vi "HH_Set.vi"(0 "Device List":T3(array[cluster]), 5 "CFD Settings":T2, 11 "error in (no error)":errorcluster, 12 "SyncDiv":i32, 13 "Offset":i32) -> (3 "ht3 header out":T1, 6 "Resolution (ps)":dbl, 8 "Range":i32, 10 "Sync Rate":i32, 15 "error out":errorcluster)   [LabVIEW 2009]
uses:
  CoreSetupNew/MT Scan/SubVIs/hhlib.dll
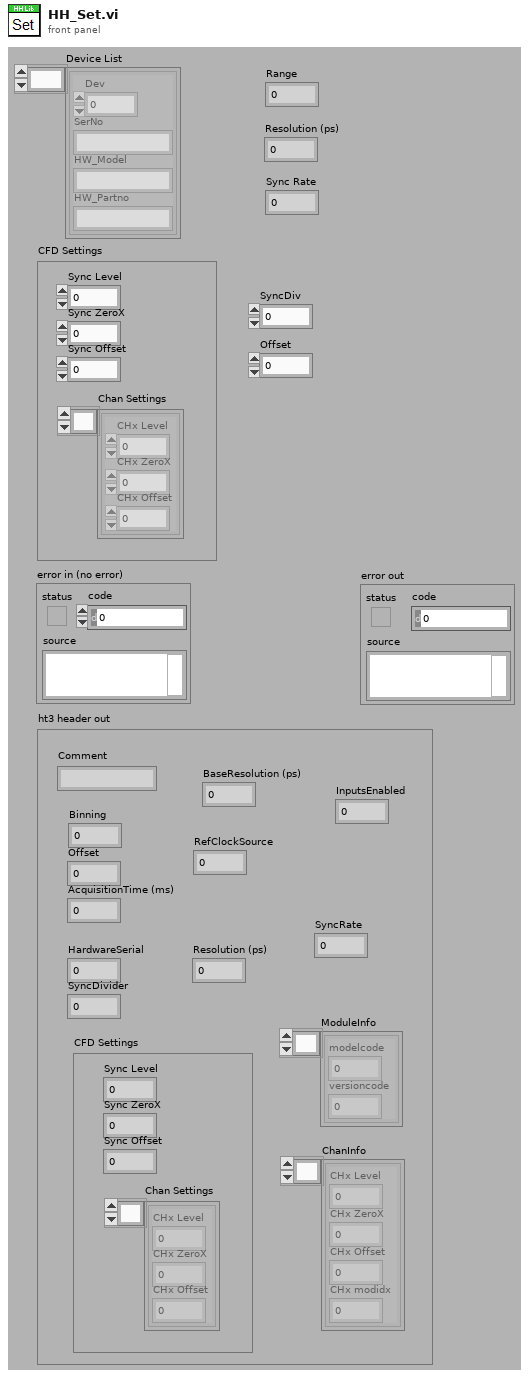
[diagram p1: front panel]
types:
  T1 = cluster{"Comment":string, "Binning":i32, "Offset":i32, "AcquisitionTime (ms)":i32, "HardwareSerial":i32, "SyncDivider":i32, "Resolution (ps)":dbl, "CFD Settings":cluster{"Sync Level":i32, "Sync ZeroX":i32, "Sync Offset":i32, "Chan Settings":cluster{"CHx Level":i32, "CHx ZeroX":i32, "CHx Offset":i32}[]}, "ModuleInfo":cluster{"modelcode":i32, "versioncode":i32}[], "BaseResolution (ps)":dbl, "RefClockSource":i32, "ChanInfo":cluster{"CHx Level":i32, "CHx ZeroX":i32, "CHx Offset":i32, "CHx modidx":i32}[], "SyncRate":i32, "InputsEnabled":i64}
  T2 = cluster{"Sync Level":i32, "Sync ZeroX":i32, "Sync Offset":i32, "Chan Settings":cluster{"CHx Level":i32, "CHx ZeroX":i32, "CHx Offset":i32}[]}
  T3 = cluster{"Dev":i32, "SerNo":string, "HW_Model":string, "HW_Partno":string}[]
  T4 = cluster{"CHx Level":i32, "CHx ZeroX":i32, "CHx Offset":i32, "CHx modidx":i32}
  T5 = cluster{"CHx Level":i32, "CHx ZeroX":i32, "CHx Offset":i32}
  T6 = cluster{"CHx Level":i32, "CHx ZeroX":i32, "CHx Offset":i32, "CHx modidx":i32}[]
  T7 = cluster{"CHx Level":i32, "CHx ZeroX":i32, "CHx Offset":i32}[]
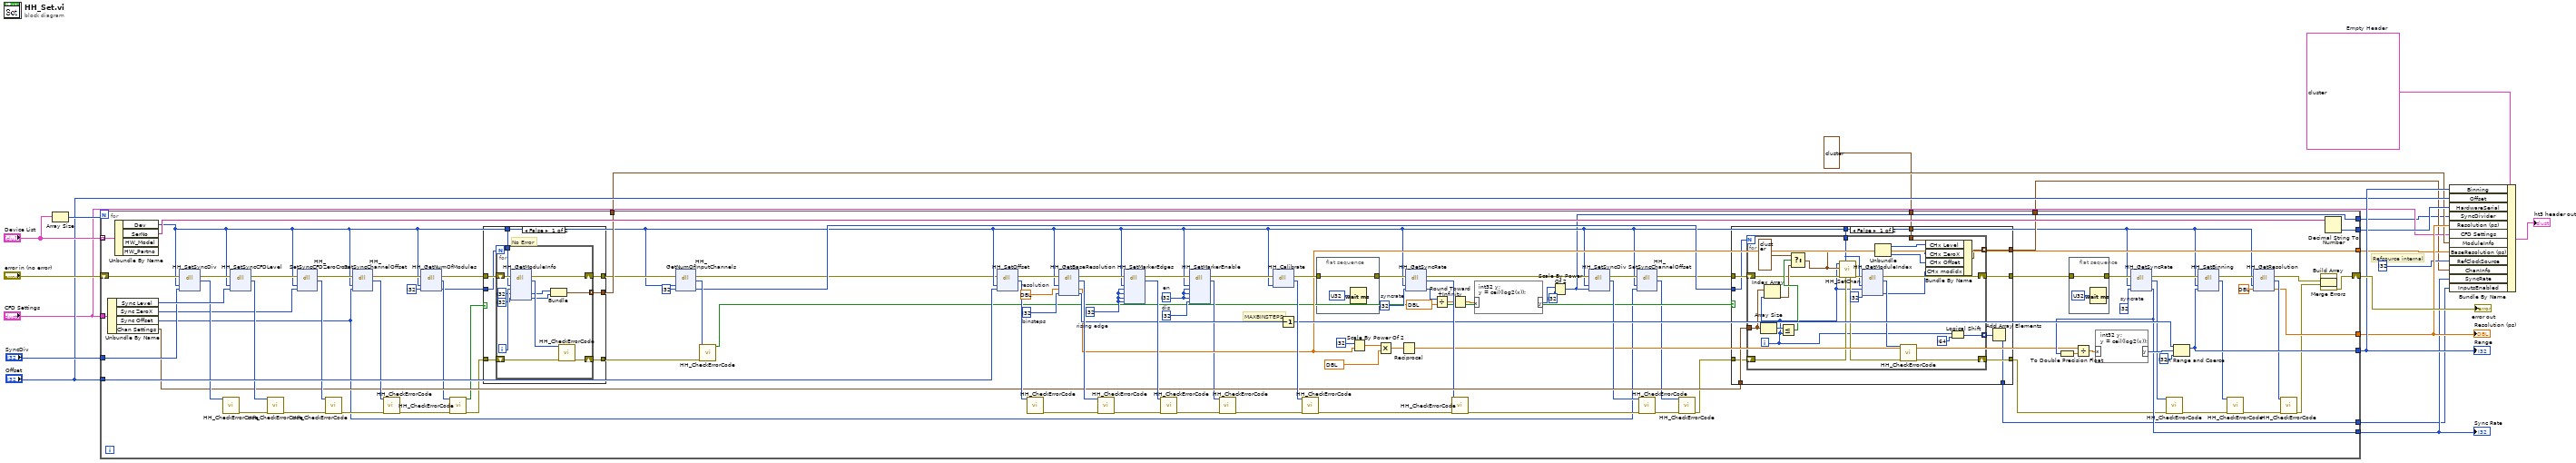
[diagram p0: block diagram]
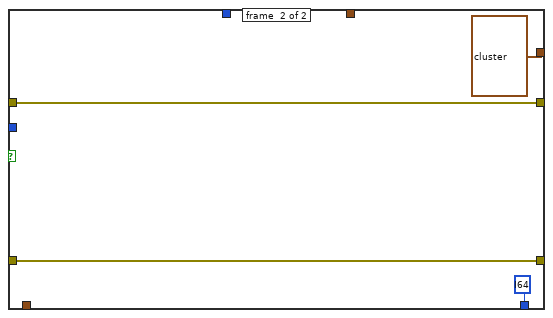
[diagram p2: hidden frame]
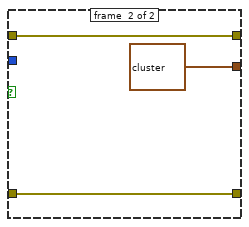
[diagram p3: hidden frame]
diagram:
  w16 = T1 ?  # Empty Header
  # "Refsource internal"
  n1 = Array Size(array="Device List") -> (size(s)=w19:i32)
  n2 = for {
    N: w19 -> [_]
    tunnel: "Device List" -> [w130] mode=indexing
    shift-right: [w94] -> w17
    shift-left: "error in (no error)" -> [w119]
    tunnel: "CFD Settings" -> [w123]
    tunnel: "SyncDiv" -> [w121]
    tunnel: "Offset" -> [w120]
    tunnel: [w112] -> w14
    tunnel: [w81] -> w10
    tunnel: [w73] -> w3
    tunnel: [w91] -> w11
    tunnel: [w53] -> w9
    tunnel: [w52] -> w8
    tunnel: [w38] -> w4
    tunnel: T4 ? ("element") -> [w37]
    tunnel: [w36] -> w2
    tunnel: [w22] -> w1
    w48 = i32 ?  # dis
    w49 = i32 ?  # en
    w74 = i32 ?  # syncrate
    w86 = i32 ?  # syncrate
    w87 = i32 ?  # binsteps
    w88 = dbl ?  # resolution
    w124 = i32 ?  # rising edge
    # "MAXBINSTEPS"
    n3 = Unbundle By Name(w123) -> ("Sync Level"=w122:i32, "Sync ZeroX"=w90:i32, "Sync Offset"=w31:i32, "Chan Settings"=w89:T7)
    n4 = Unbundle By Name(w130) -> ("Dev"=w32:i32, "SerNo"=w92:string)  [unwired: 2 out]
    n5 = dll-call lib="C:/Users/dhaehnel/Documents/Workspace/Labview_Workspace/CoreSetupNew/MT Scan/SubVIs/hhlib.dll" fn="HH_SetSyncDiv"(error in=w119, "devidx"=w32, "div"=w121) -> (error out=w129:errorcluster, "return type"=w110:i32)  [unwired: 4 in, 1 out]
    n6 = call "HH_CheckErrorCode.vi"("errcode"=w110) -> ("error out"=w109:errorcluster)  [unwired: 13 in, 1 out]
    n7 = dll-call lib="C:/Users/dhaehnel/Documents/Workspace/Labview_Workspace/CoreSetupNew/MT Scan/SubVIs/hhlib.dll" fn="HH_SetSyncCFDLevel"(error in=w129, "devidx"=w32, "value"=w122) -> (error out=w128:errorcluster, "return type"=w108:i32)  [unwired: 4 in, 1 out]
    n8 = call "HH_CheckErrorCode.vi"("errcode"=w108, "error in (no error)"=w109) -> ("error out"=w107:errorcluster)  [unwired: 12 in, 1 out]
    n9 = dll-call lib="C:/Users/dhaehnel/Documents/Workspace/Labview_Workspace/CoreSetupNew/MT Scan/SubVIs/hhlib.dll" fn="HH_SetSyncCFDZeroCross" label="HH_SetSyncZeroX"(error in=w128, "devidx"=w32, "value"=w90) -> (error out=w127:errorcluster, "return type"=w106:i32)  [unwired: 4 in, 1 out]
    n10 = call "HH_CheckErrorCode.vi"("errcode"=w106, "error in (no error)"=w107) -> ("error out"=w104:errorcluster)  [unwired: 12 in, 1 out]
    n11 = dll-call lib="C:/Users/dhaehnel/Documents/Workspace/Labview_Workspace/CoreSetupNew/MT Scan/SubVIs/hhlib.dll" fn="HH_SetSyncChannelOffset" label="HH_SetSyncChOffset"(error in=w127, "devidx"=w32, "value"=w31) -> (error out=w55:errorcluster, "return type"=w105:i32)  [unwired: 4 in, 1 out]
    n12 = call "HH_CheckErrorCode.vi"("errcode"=w105, "error in (no error)"=w104) -> ("error out"=w56:errorcluster)  [unwired: 12 in, 1 out]
    n13 = dll-call lib="C:/Users/dhaehnel/Documents/Workspace/Labview_Workspace/CoreSetupNew/MT Scan/SubVIs/hhlib.dll" fn="HH_GetNumOfModules"(error in=w55, "devidx"=w32, "nummod"=i32 ?) -> (error out=w58:errorcluster, "return type"=w60:i32, "nummod"=w57:i32)  [unwired: 3 in, 1 out]
    n14 = call "HH_CheckErrorCode.vi"("errcode"=w60, "error in (no error)"=w56) -> ("Is Error"=w59:bool, "error out"=w54:errorcluster)  [unwired: 12 in]
    n15 = case shown="False" w59 {
      tunnel: w58 -> [w176 w191]
      tunnel: [w175 w191] -> w44
      tunnel: w57 -> [w174 _]
      tunnel: w54 -> [w173 w190]
      tunnel: [w172 w190] -> w43
      tunnel: w32 -> [w171 _]
      tunnel: [w170 cluster{"modelcode":i32, "versioncode":i32}[] ?] -> w53
      frame #0 {
        # "No Error"
        n16 = for {
          N: w174 -> [_]
          shift-right: [w180] -> w175
          shift-left: w176 -> [w188]
          shift-right: [w186] -> w172
          shift-left: w173 -> [w187]
          tunnel: w171 -> [w184]
          tunnel: [w177] -> w170 mode=indexing
          i -> [w183]
          n17 = dll-call lib="C:/Users/dhaehnel/Documents/Workspace/Labview_Workspace/CoreSetupNew/MT Scan/SubVIs/hhlib.dll" fn="HH_GetModuleInfo"(error in=w188, "devidx"=w184, "modidx"=w183, "modelcode"=i32 ?, "versioncode"=i32 ?) -> (error out=w180:errorcluster, "return type"=w185:i32, "modelcode"=w179:i32, "versioncode"=w178:i32)  [unwired: 4 in, 1 out]
          n18 = Bundle("modelcode"=w179, "versioncode"=w178) -> (w177:cluster{"modelcode":i32, "versioncode":i32})  [unwired: 1 in]
          n19 = call "HH_CheckErrorCode.vi"("errcode"=w185, "error in (no error)"=w187) -> ("error out"=w186:errorcluster)  [unwired: 12 in, 1 out]
        }
      }
      frame #1 {
      }
    }
    n20 = dll-call lib="C:/Users/dhaehnel/Documents/Workspace/Labview_Workspace/CoreSetupNew/MT Scan/SubVIs/hhlib.dll" fn="HH_GetNumOfInputChannels"(error in=w44, "devidx"=w32, "nchannels"=i32 ?) -> (error out=w26:errorcluster, "return type"=w42:i32, "nchannels"=w39:i32)  [unwired: 3 in, 1 out]
    n21 = call "HH_CheckErrorCode.vi"("errcode"=w42, "error in (no error)"=w43) -> ("Is Error"=w41:bool)  [unwired: 12 in, 1 out]
    n22 = dll-call lib="C:/Users/dhaehnel/Documents/Workspace/Labview_Workspace/CoreSetupNew/MT Scan/SubVIs/hhlib.dll" fn="HH_SetOffset"(error in=w26, "devidx"=w32, "offset"=w120) -> (error out=w126:errorcluster, "return type"=w103:i32)  [unwired: 4 in, 1 out]
    n23 = call "HH_CheckErrorCode.vi"("errcode"=w103) -> ("error out"=w102:errorcluster)  [unwired: 13 in, 1 out]
    n24 = dll-call lib="C:/Users/dhaehnel/Documents/Workspace/Labview_Workspace/CoreSetupNew/MT Scan/SubVIs/hhlib.dll" fn="HH_GetBaseResolution"(error in=w126, "devidx"=w32, "resolution"=w88, "binsteps"=w87) -> (error out=w125:errorcluster, "return type"=w93:i32, "resolution"=w52:dbl, "binsteps"=w84:i32)  [unwired: 3 in, 1 out]
    n25 = call "HH_CheckErrorCode.vi"("errcode"=w93, "error in (no error)"=w102) -> ("error out"=w101:errorcluster)  [unwired: 12 in, 1 out]
    n26 = dll-call lib="C:/Users/dhaehnel/Documents/Workspace/Labview_Workspace/CoreSetupNew/MT Scan/SubVIs/hhlib.dll" fn="HH_SetMarkerEdges"(error in=w125, "devidx"=w32, "me0"=w124, "me1"=w124, "me2"=w124, "me3"=w124) -> (error out=w51:errorcluster, "return type"=w100:i32)  [unwired: 7 in, 1 out]
    n27 = call "HH_CheckErrorCode.vi"("errcode"=w100, "error in (no error)"=w101) -> ("error out"=w47:errorcluster)  [unwired: 12 in, 1 out]
    n28 = dll-call lib="C:/Users/dhaehnel/Documents/Workspace/Labview_Workspace/CoreSetupNew/MT Scan/SubVIs/hhlib.dll" fn="HH_SetMarkerEnable"(error in=w51, "devidx"=w32, "en0"=w49, "en1"=w49, "en2"=w49, "en3"=w48) -> (error out=w50:errorcluster, "return type"=w45:i32)  [unwired: 7 in, 1 out]
    n29 = call "HH_CheckErrorCode.vi"("errcode"=w45, "error in (no error)"=w47) -> ("error out"=w46:errorcluster)  [unwired: 12 in, 1 out]
    n30 = dll-call lib="C:/Users/dhaehnel/Documents/Workspace/Labview_Workspace/CoreSetupNew/MT Scan/SubVIs/hhlib.dll" fn="HH_Calibrate"(error in=w50, "devidx"=w32) -> (error out=w118:errorcluster, "return type"=w99:i32)  [unwired: 3 in, 1 out]
    n31 = Decrement(x=w84) -> (x-1=w83:i32)
    n32 = call "HH_CheckErrorCode.vi"("errcode"=w99, "error in (no error)"=w46) -> ("error out"=w98:errorcluster)  [unwired: 12 in, 1 out]
    n33 = flat-sequence {
      tunnel: w118 -> [w195]
      tunnel: [w195] -> w117
      frame #0 {
        n34 = Wait (ms)(milliseconds to wait=u32 ?) -> ()  [unwired: 1 out]
      }
    }
    n35 = Scale By Power Of 2(n=i32 ?, x=w52) -> (x*2^n=w67:dbl)
    n36 = Multiply(x=w67, y=dbl ?) -> (x*y=w65:dbl)
    n37 = Reciprocal(x=w65) -> (1/x=w64:dbl)
    n38 = dll-call lib="C:/Users/dhaehnel/Documents/Workspace/Labview_Workspace/CoreSetupNew/MT Scan/SubVIs/hhlib.dll" fn="HH_GetSyncRate"(error in=w117, "devidx"=w32, "syncrate"=w86) -> (error out=w80:errorcluster, "return type"=w85:i32, "syncrate"=w79:i32)  [unwired: 3 in, 1 out]
    n39 = Divide(x=w79, y=dbl ?) -> (x/y=w77:dbl)
    n40 = call "HH_CheckErrorCode.vi"("errcode"=w85, "error in (no error)"=w98) -> ("error out"=w70:errorcluster)  [unwired: 12 in, 1 out]
    n41 = Round Toward +Infinity(x=w77) -> (ceil(x): smallest int >= x=w25:dbl)
    n42 = formula code="int32 y;\ny = ceil(log2(x));"("x"=w25) -> ("y"=w24:i32)
    n43 = Scale By Power Of 2(n=w24, x=i32 ?) -> (x*2^n=w22:i32)
    n44 = dll-call lib="C:/Users/dhaehnel/Documents/Workspace/Labview_Workspace/CoreSetupNew/MT Scan/SubVIs/hhlib.dll" fn="HH_SetSyncDiv"(error in=w80, "devidx"=w32, "div"=w22) -> (error out=w35:errorcluster, "return type"=w72:i32)  [unwired: 4 in, 1 out]
    n45 = dll-call lib="C:/Users/dhaehnel/Documents/Workspace/Labview_Workspace/CoreSetupNew/MT Scan/SubVIs/hhlib.dll" fn="HH_SetSyncChannelOffset" label="HH_SetSyncChOffset"(error in=w35, "devidx"=w32, "value"=w31) -> (error out=w27:errorcluster, "return type"=w33:i32)  [unwired: 4 in, 1 out]
    n46 = call "HH_CheckErrorCode.vi"("errcode"=w72, "error in (no error)"=w70) -> ("error out"=w34:errorcluster)  [unwired: 12 in, 1 out]
    n47 = call "HH_CheckErrorCode.vi"("errcode"=w33, "error in (no error)"=w34) -> ("error out"=w30:errorcluster)  [unwired: 12 in, 1 out]
    n48 = case shown="False" w41 {
      tunnel: w89 -> [w141 _]
      tunnel: [w140 w169] -> w28
      tunnel: [w139 w168] -> w29
      tunnel: w27 -> [w138 w169]
      tunnel: w32 -> [w137 _]
      tunnel: w30 -> [w136 w168]
      tunnel: w39 -> [w135 _]
      tunnel: [w134 T6 ?] -> w38
      tunnel: w37 -> [w133 _]
      tunnel: [w131 i64 ?] -> w36
      frame #0 {
        n49 = for {
          N: w135 -> [_]
          tunnel: w141 -> [w164]
          tunnel: w137 -> [w156]
          shift-right: [w157] -> w140
          shift-left: w138 -> [w160]
          shift-right: [w153] -> w139
          shift-left: w136 -> [w159]
          tunnel: [w150] -> w134 mode=indexing
          tunnel: w133 -> [w151]
          tunnel: [w142] -> w132 mode=indexing
          i -> [w144]
          n50 = Array Size(array=w164) -> (size(s)=w165:i32)
          n51 = Index Array(array=w164, index=w144) -> (element=w161:T5)
          n52 = Less Or Equal?(x=w165, y=w144) -> (x <= y?=w163:bool)
          n53 = Select(t=T5 ? ("element"), s=w163, f=w161) -> (s? t:f=w148:T5)
          n54 = call "HH_SetChan.vi"("error in 2"=w159, "Dev"=w156, "error in"=w160, "CHx CFD Settings"=w148, "Chan"=w144) -> ("error out"=w158:errorcluster, "error out 2"=w154:errorcluster)  [unwired: 5 in]
          n55 = dll-call lib="C:/Users/dhaehnel/Documents/Workspace/Labview_Workspace/CoreSetupNew/MT Scan/SubVIs/hhlib.dll" fn="HH_GetModuleIndex"(error in=w158, "devidx"=w156, "channel"=w144, "modidx"=i32 ?) -> (error out=w157:errorcluster, "return type"=w152:i32, "modidx"=w149:i32)  [unwired: 4 in, 1 out]
          n56 = Unbundle(w148) -> ("CHx Level"=w147:i32, "CHx ZeroX"=w145:i32, "CHx Offset"=w146:i32)
          n57 = call "HH_CheckErrorCode.vi"("errcode"=w152, "error in (no error)"=w154) -> ("error out"=w153:errorcluster)  [unwired: 12 in, 1 out]
          n58 = Bundle By Name(cluster=w151, "CHx Level"=w147, "CHx ZeroX"=w145, "CHx Offset"=w146, "CHx modidx"=w149) -> (w150:T4)
          n59 = Logical Shift(y=w144, x=i64 ?) -> (x << y=w142:i64)
        }
        n60 = Add Array Elements(numeric array=w132) -> (sum=w131:i64)
      }
      frame #1 {
      }
    }
    n61 = flat-sequence {
      tunnel: w28 -> [w193]
      tunnel: [w193] -> w76
      frame #0 {
        n62 = Wait (ms)(milliseconds to wait=u32 ?) -> ()  [unwired: 1 out]
      }
    }
    n63 = dll-call lib="C:/Users/dhaehnel/Documents/Workspace/Labview_Workspace/CoreSetupNew/MT Scan/SubVIs/hhlib.dll" fn="HH_GetSyncRate"(error in=w76, "devidx"=w32, "syncrate"=w74) -> (error out=w75:errorcluster, "return type"=w71:i32, "syncrate"=w73:i32)  [unwired: 3 in, 1 out]
    n64 = To Double Precision Float(number=w73) -> (double precision float=w114:dbl)
    n65 = Divide(x=w64, y=w114) -> (x/y=w116:dbl)
    n66 = formula code="int32 y;\ny = ceil(log2(x));"("x"=w116) -> ("y"=w113:i32)
    n67 = call "HH_CheckErrorCode.vi"("errcode"=w71, "error in (no error)"=w29) -> ("error out"=w69:errorcluster)  [unwired: 12 in, 1 out]
    n68 = In Range and Coerce(upper limit=w83, x=w113, lower limit=i32 ?) -> (coerced(x)=w112:i32)  [unwired: 1 out]
    n69 = dll-call lib="C:/Users/dhaehnel/Documents/Workspace/Labview_Workspace/CoreSetupNew/MT Scan/SubVIs/hhlib.dll" fn="HH_SetBinning"(error in=w75, "devidx"=w32, "binning"=w112) -> (error out=w115:errorcluster, "return type"=w97:i32)  [unwired: 4 in, 1 out]
    n70 = call "HH_CheckErrorCode.vi"("errcode"=w97, "error in (no error)"=w69) -> ("error out"=w96:errorcluster)  [unwired: 12 in, 1 out]
    n71 = dll-call lib="C:/Users/dhaehnel/Documents/Workspace/Labview_Workspace/CoreSetupNew/MT Scan/SubVIs/hhlib.dll" fn="HH_GetResolution"(error in=w115, "devidx"=w32, "resolution"=dbl ?) -> (error out=w63:errorcluster, "return type"=w95:i32, "resolution"=w81:dbl)  [unwired: 3 in, 1 out]
    n72 = call "HH_CheckErrorCode.vi"("errcode"=w95, "error in (no error)"=w96) -> ("error out"=w62:errorcluster)  [unwired: 12 in, 1 out]
    n73 = Build Array(w63, w62) -> (w21:errorcluster[])
    n74 = call <vilib>:"Merge Errors.vi"("error array in"=w21) -> ("error out"=w94:errorcluster)  [unwired: 6 in]
    n75 = Decimal String To Number(string=w92) -> (number=w91:i32)  [unwired: 2 in, 1 out]
  }
  "error out" <- w17
  "Range" <- w14
  "Resolution (ps)" <- w10
  "Sync Rate" <- w3
  n76 = Bundle By Name(cluster=w16, "Binning"=w14, "Offset"="Offset", "HardwareSerial"=w11, "SyncDivider"=w1, "Resolution (ps)"=w10, "CFD Settings"="CFD Settings", "ModuleInfo"=w9, "BaseResolution (ps)"=w8, "RefClockSource"=i32 ? ("refsource"), "ChanInfo"=w4, "SyncRate"=w3, "InputsEnabled"=w2) -> (→"ht3 header out":T1)
